vi "SV UFF58 Format ASCII Ordinate Data (Evenly Spaced).vi"(6 "ordinate data type":u16(ring)=6 items=["real single precision"=2, "real double precision"=4, "complex single precision"=5, "complex double precision"=6], 8 "ordinate values (Y Im)":dbl[](array[numeric]), 9 "ordinate values (Y Re)":dbl[](array[numeric]), 11 "formatted UFF58 ASCII header":string) -> (3 "UFF58 ASCII function string":string)   [LabVIEW 2017, in "SoundVib_UFF58.lvlib"]
doc: "Formats record 12 to the UFF58 (universal file format) ASCII data format. The input <B>formatted UFF58 ASCII header</B> string concatenates with the formatted data and is returned in the UFF58 ASCII function string. You also can use this VI in combination with the SVT UFF58 Read VI to convert UFF58 function data from binary to ASCII format."
uses:
  <vilib>/addons/Sound and Vibration/svt_UFF58/SoundVib_UFF58.lvlib
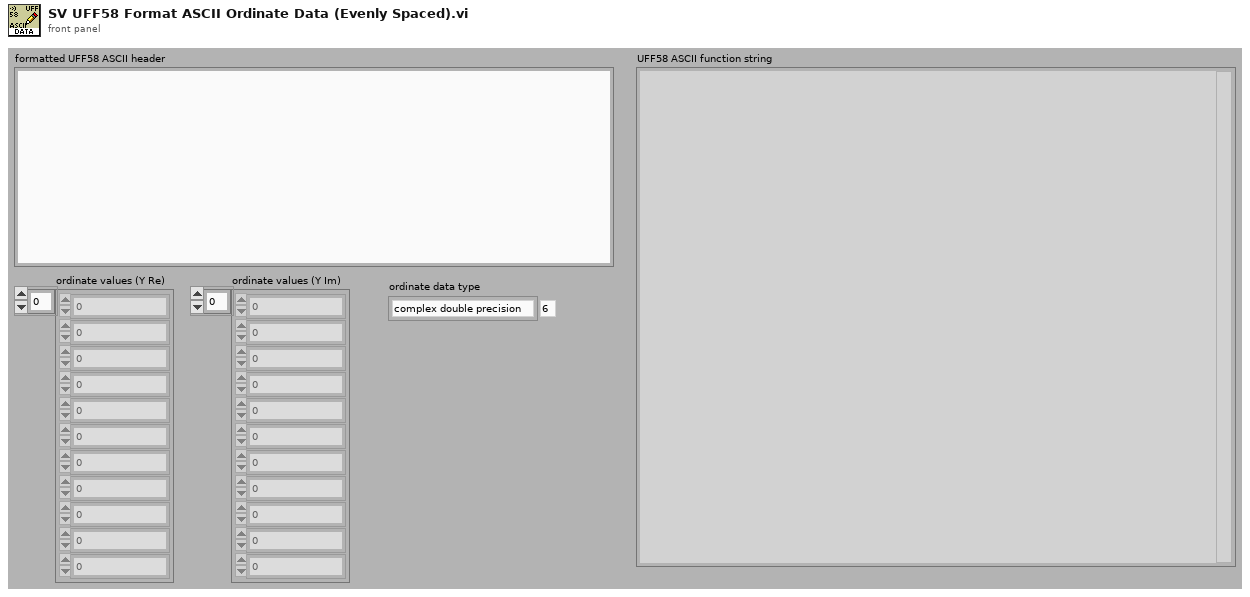
[diagram p1: front panel]
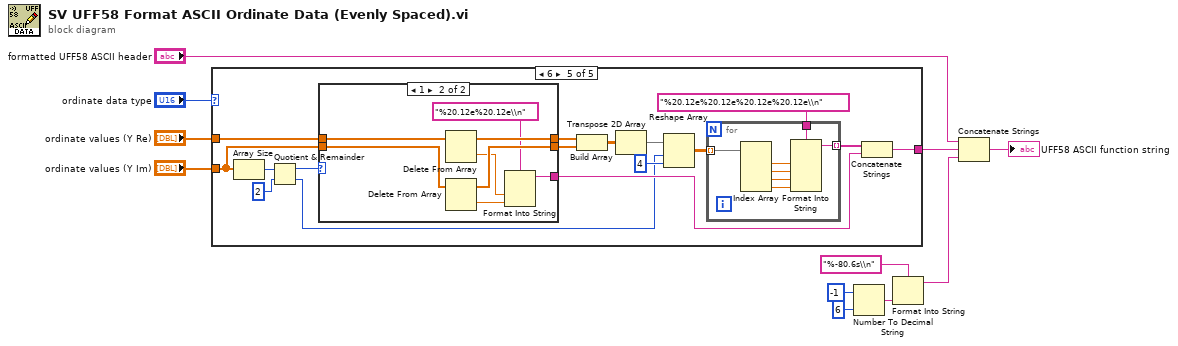
[diagram p0: block diagram]
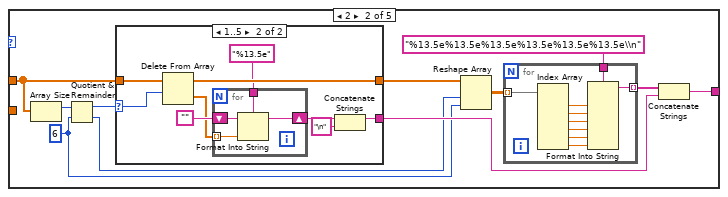
[diagram p3: hidden frame]
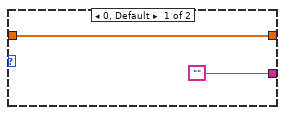
[diagram p4: hidden frame]
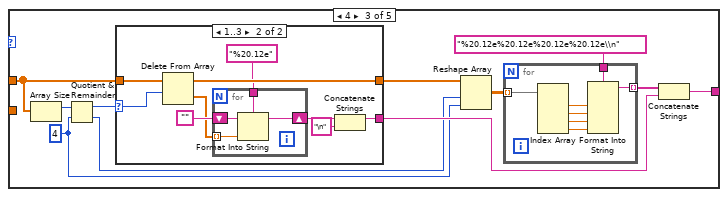
[diagram p5: hidden frame]
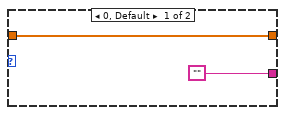
[diagram p6: hidden frame]
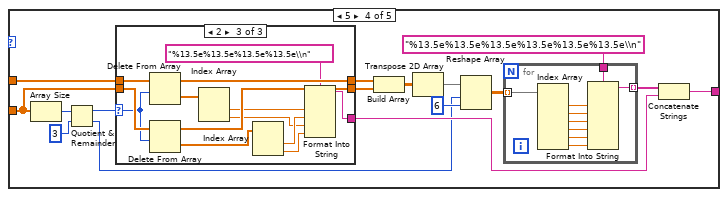
[diagram p7: hidden frame]
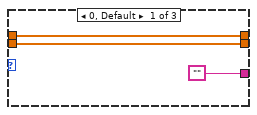
[diagram p8: hidden frame]
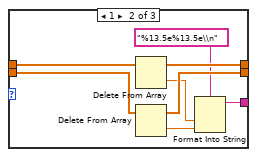
[diagram p9: hidden frame]
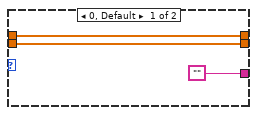
[diagram p10: hidden frame]
diagram:
  n1 = case shown="6" "ordinate data type" {
    tunnel: [_ w15 w50 w82 w131] -> w10
    tunnel: "ordinate values (Y Re)" -> [_ w12 w47 w81 w130]
    tunnel: "ordinate values (Y Im)" -> [_ _ _ w80 w129]
    frame 0, Default {
    }
    frame 2 {
      w13 = 6 ("y")
      n2 = Array Size(array=w12) -> (size(s)=w22:i32)
      n3 = Quotient & Remainder(x=w22, y=w13) -> (x-y*floor(x/y)=w21:i32, floor(x/y)=w16:i32)
      n4 = case shown="1..5" w21 {
        selector: w21 -> [_ w39]
        tunnel: w12 -> [w33 w42]
        tunnel: [w33 w41] -> w14
        tunnel: ["" w35] -> w17
        frame 0, Default {
        }
        frame 1..5 {
          n5 = Delete From Array(array=w42, length=w39) -> (deleted portion=w37:dbl[], array with subset deleted=w41:dbl[])  [unwired: 1 in]
          n6 = for {
            tunnel: "%13.5e" ("format string") -> [w46]
            shift-right: [w45] -> w36
            shift-left: "" -> [w44]
            tunnel: w37 -> [w43] mode=indexing
            n7 = Format Into String(format string=w46, initial string=w44, w43) -> (resulting string=w45:string)  [unwired: 1 in, 1 out]
          }
          n8 = Concatenate Strings(w36, "\n" ("string")) -> (w35:string)
        }
      }
      n9 = Reshape Array(w14, w16, w13) -> (w20:dbl[][])
      n10 = for {
        tunnel: w20 -> [w31] mode=indexing
        tunnel: "%13.5e%13.5e%13.5e%13.5e%13.5e%13.5e\\n" ("format string") -> [w26]
        tunnel: [w25] -> w18 mode=indexing
        n11 = Index Array(array=w31) -> (element #1=w30:dbl, element #2=w29:dbl, element #3=w28:dbl, element #4=w27:dbl, element #5=w24:dbl, element #6=w23:dbl)  [unwired: 6 in]
        n12 = Format Into String(format string=w26, w30, w29, w28, w27, w24, w23) -> (resulting string=w25:string)  [unwired: 2 in, 1 out]
      }
      n13 = Concatenate Strings(w18, w17) -> (w15:string)
    }
    frame 4 {
      w48 = 4 ("y")
      n14 = Array Size(array=w47) -> (size(s)=w57:i32)
      n15 = Quotient & Remainder(x=w57, y=w48) -> (x-y*floor(x/y)=w56:i32, floor(x/y)=w51:i32)
      n16 = case shown="1..3" w56 {
        selector: w56 -> [_ w72]
        tunnel: w47 -> [w66 w75]
        tunnel: [w66 w74] -> w49
        tunnel: ["" w68] -> w52
        frame 0, Default {
        }
        frame 1..3 {
          n17 = Delete From Array(array=w75, length=w72) -> (deleted portion=w70:dbl[], array with subset deleted=w74:dbl[])  [unwired: 1 in]
          n18 = for {
            tunnel: "%20.12e" ("format string") -> [w79]
            shift-right: [w78] -> w69
            shift-left: "" -> [w77]
            tunnel: w70 -> [w76] mode=indexing
            n19 = Format Into String(format string=w79, initial string=w77, w76) -> (resulting string=w78:string)  [unwired: 1 in, 1 out]
          }
          n20 = Concatenate Strings(w69, "\n" ("string")) -> (w68:string)
        }
      }
      n21 = Reshape Array(w49, w51, w48) -> (w55:dbl[][])
      n22 = for {
        tunnel: w55 -> [w64] mode=indexing
        tunnel: "%20.12e%20.12e%20.12e%20.12e\\n" ("format string") -> [w59]
        tunnel: [w58] -> w53 mode=indexing
        n23 = Index Array(array=w64) -> (element #1=w63:dbl, element #2=w62:dbl, element #3=w61:dbl, element #4=w60:dbl)  [unwired: 4 in]
        n24 = Format Into String(format string=w59, w63, w62, w61, w60) -> (resulting string=w58:string)  [unwired: 2 in, 1 out]
      }
      n25 = Concatenate Strings(w53, w52) -> (w50:string)
    }
    frame 5 {
      n26 = Array Size(array=w80) -> (size(s)=w94:i32)
      n27 = Quotient & Remainder(x=w94, y=3) -> (x-y*floor(x/y)=w88:i32, floor(x/y)=w83:i32)
      n28 = case shown="2" w88 {
        selector: w88 -> [_ _ w121]
        tunnel: w80 -> [w106 w115 w128]
        tunnel: [w106 w114 w127] -> w90
        tunnel: w81 -> [w107 w113 w126]
        tunnel: [w107 w112 w125] -> w89
        tunnel: ["" w108 w122] -> w84
        frame 0, Default {
        }
        frame 1 {
          n29 = Delete From Array(array=w113) -> (deleted portion=w110:dbl, array with subset deleted=w112:dbl[])  [unwired: 2 in]
          n30 = Delete From Array(array=w115) -> (deleted portion=w109:dbl, array with subset deleted=w114:dbl[])  [unwired: 2 in]
          n31 = Format Into String(format string="%13.5e%13.5e\\n", w110, w109) -> (resulting string=w108:string)  [unwired: 2 in, 1 out]
        }
        frame 2 {
          n32 = Delete From Array(array=w126, length=w121) -> (deleted portion=w123:dbl[], array with subset deleted=w125:dbl[])  [unwired: 1 in]
          n33 = Delete From Array(array=w128, length=w121) -> (deleted portion=w119:dbl[], array with subset deleted=w127:dbl[])  [unwired: 1 in]
          n34 = Index Array(array=w123) -> (element #1=w120:dbl, element #2=w116:dbl)  [unwired: 2 in]
          n35 = Index Array(array=w119) -> (element #1=w118:dbl, element #2=w117:dbl)  [unwired: 2 in]
          n36 = Format Into String(format string="%13.5e%13.5e%13.5e%13.5e\\n", w120, w118, w116, w117) -> (resulting string=w122:string)  [unwired: 2 in, 1 out]
        }
      }
      n37 = Build Array(w89, w90) -> (w95:dbl[][])
      n38 = Transpose 2D Array(2D array=w95) -> (transposed array=w92:dbl[][])
      n39 = Reshape Array(w92, w83, 6 ("dimension size")) -> (w87:dbl[][])
      n40 = for {
        tunnel: w87 -> [w104] mode=indexing
        tunnel: "%13.5e%13.5e%13.5e%13.5e%13.5e%13.5e\\n" ("format string") -> [w99]
        tunnel: [w98] -> w85 mode=indexing
        n41 = Index Array(array=w104) -> (element #1=w103:dbl, element #2=w102:dbl, element #3=w101:dbl, element #4=w100:dbl, element #5=w97:dbl, element #6=w96:dbl)  [unwired: 6 in]
        n42 = Format Into String(format string=w99, w103, w102, w101, w100, w97, w96) -> (resulting string=w98:string)  [unwired: 2 in, 1 out]
      }
      n43 = Concatenate Strings(w85, w84) -> (w82:string)
    }
    frame 6 {
      n44 = Array Size(array=w129) -> (size(s)=w143:i32)
      n45 = Quotient & Remainder(x=w143, y=2) -> (x-y*floor(x/y)=w137:i32, floor(x/y)=w132:i32)
      n46 = case shown="1" w137 {
        tunnel: w129 -> [w153 w162]
        tunnel: [w153 w161] -> w139
        tunnel: w130 -> [w154 w160]
        tunnel: [w154 w159] -> w138
        tunnel: ["" w155] -> w133
        frame 0, Default {
        }
        frame 1 {
          n47 = Delete From Array(array=w160) -> (deleted portion=w157:dbl, array with subset deleted=w159:dbl[])  [unwired: 2 in]
          n48 = Delete From Array(array=w162) -> (deleted portion=w156:dbl, array with subset deleted=w161:dbl[])  [unwired: 2 in]
          n49 = Format Into String(format string="%20.12e%20.12e\\n", w157, w156) -> (resulting string=w155:string)  [unwired: 2 in, 1 out]
        }
      }
      n50 = Build Array(w138, w139) -> (w144:dbl[][])
      n51 = Transpose 2D Array(2D array=w144) -> (transposed array=w141:dbl[][])
      n52 = Reshape Array(w141, w132, 4 ("dimension size")) -> (w136:dbl[][])
      n53 = for {
        tunnel: w136 -> [w151] mode=indexing
        tunnel: "%20.12e%20.12e%20.12e%20.12e\\n" ("format string") -> [w146]
        tunnel: [w145] -> w134 mode=indexing
        n54 = Index Array(array=w151) -> (element #1=w150:dbl, element #2=w149:dbl, element #3=w148:dbl, element #4=w147:dbl)  [unwired: 4 in]
        n55 = Format Into String(format string=w146, w150, w149, w148, w147) -> (resulting string=w145:string)  [unwired: 2 in, 1 out]
      }
      n56 = Concatenate Strings(w134, w133) -> (w131:string)
    }
  }
  n57 = Number To Decimal String(number=-1, width (-)=i16 6) -> (decimal integer string=w4:string)
  n58 = Format Into String(format string="%-80.6s\\n", w4) -> (resulting string=w8:string)  [unwired: 2 in, 1 out]
  n59 = Concatenate Strings("formatted UFF58 ASCII header", w10, w8) -> (→"UFF58 ASCII function string":string)
